vi "command_line_args.vi"(8 "error in (no error)":errorcluster, 10 "App.Args":string[](array[string]), 11 "Message Queues In":T1) -> (0 "error out":errorcluster, 2 "2D Array":string[][](array[string]), 3 "Message Queues Out":T1)   [LabVIEW 2013]
doc: "Receives the Command Line Arguments provided when the application was executed. The commands are decoded and translated to GUI sequence of GUI states for Main.vis"
uses:
  queues/que_all_message_queues.ctl
  queues/que_message_cluster.ctl
  type_def/general.ctl
  queues/que_enqueue_message_single.vi
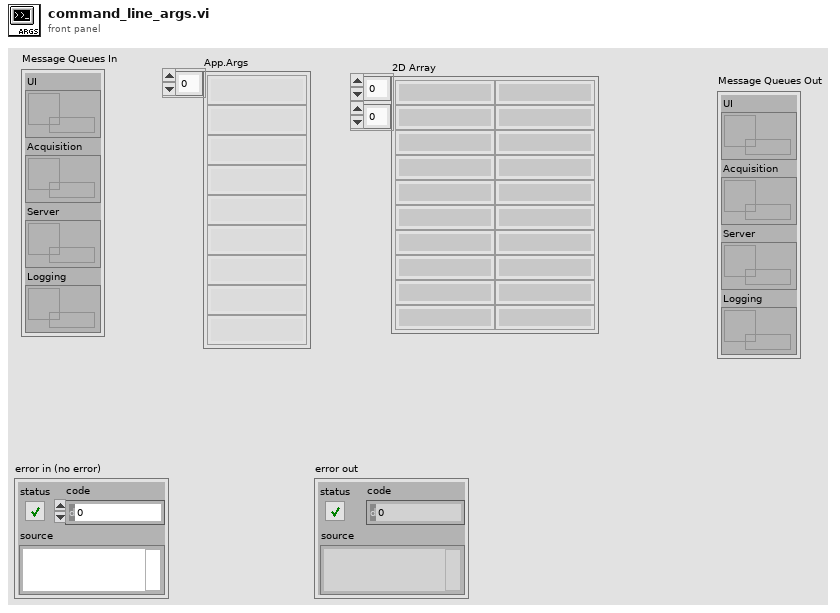
[diagram p1: front panel]
types:
  T1 = typedef "que_all_message_queues.ctl" = cluster{"UI":refnum<queue>, "Acquisition":refnum<queue>, "Server":refnum<queue>, "Logging":refnum<queue>}
  T2 = typedef "general.ctl" = cluster{"file_ext":string, "TCP port":i32, "#devices":i32, "log?":bool, "tcp?":bool, "language":string}
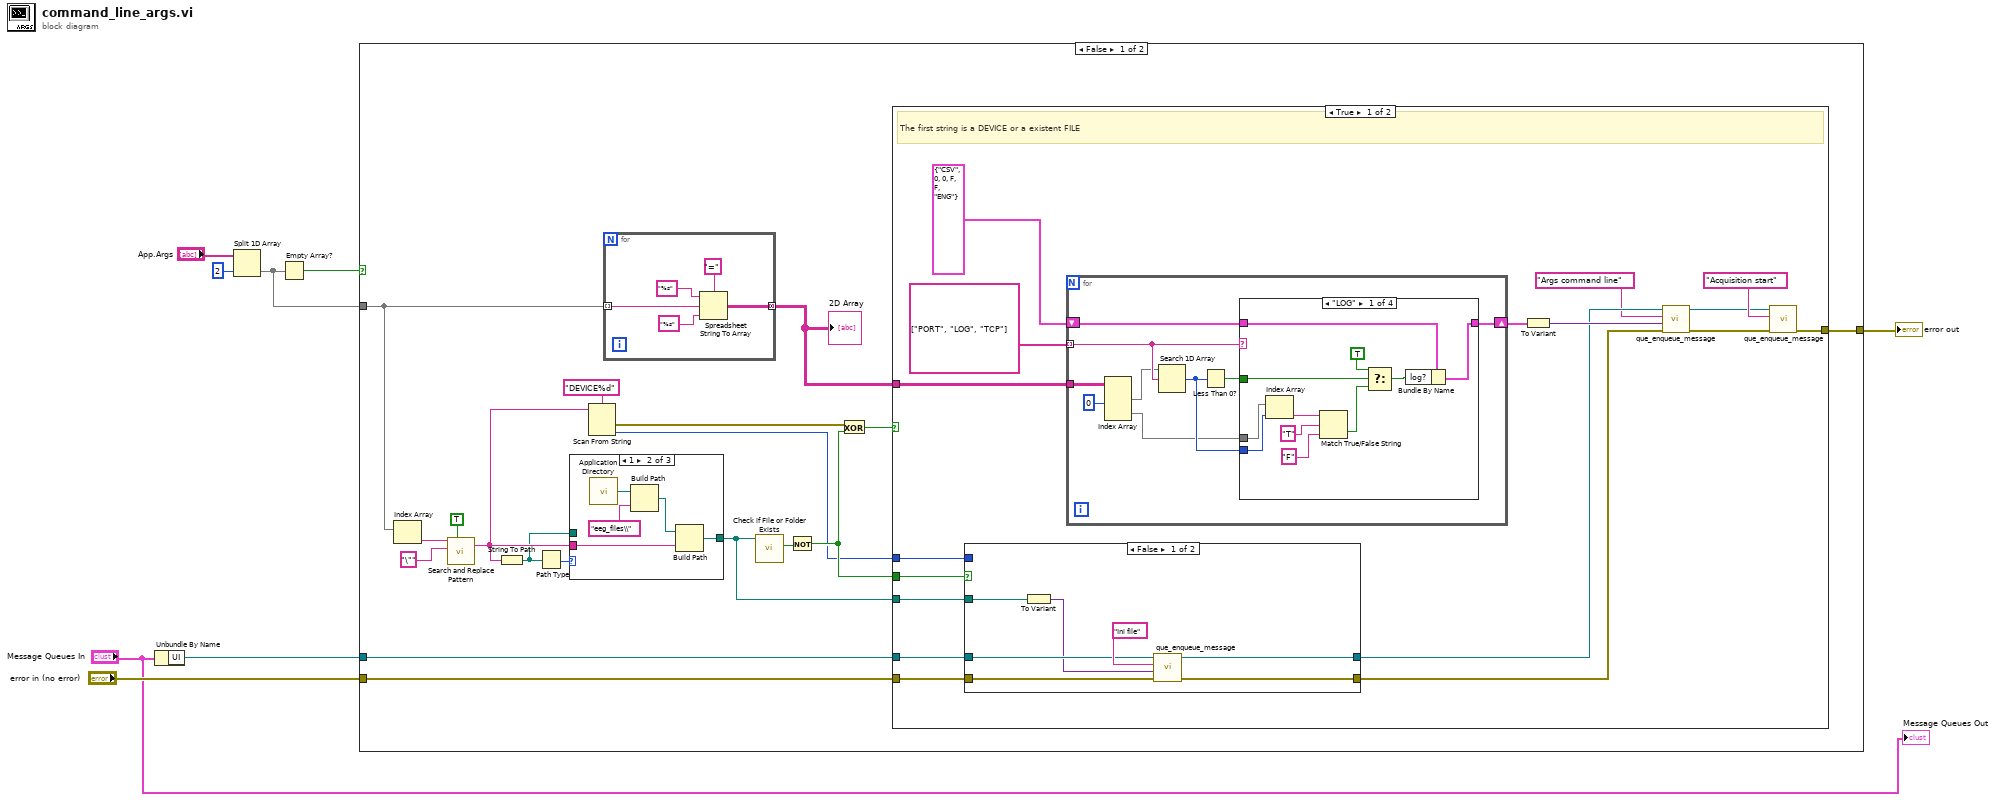
[diagram p0: block diagram]
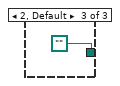
[diagram p3: hidden frame]
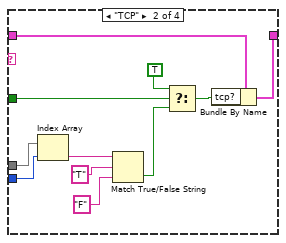
[diagram p4: hidden frame]
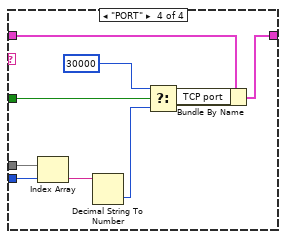
[diagram p6: hidden frame]
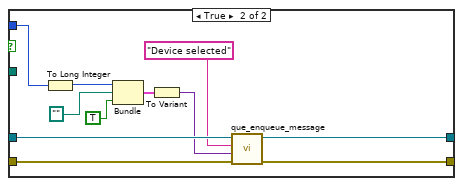
[diagram p7: hidden frame]
diagram:
  n1 = Unbundle By Name("Message Queues In") -> ("UI"=w2:refnum<queue>)
  n2 = Split 1D Array(array="App.Args", index=2) -> (second subarray=w4:string[])  [unwired: 1 out]
  n3 = Empty Array?(array=w4) -> (empty?=w5:bool)
  n4 = case shown="False" w5 {
    tunnel: [w26 w116] -> w8
    tunnel: "error in (no error)" -> [w9 w116]
    tunnel: w2 -> [w10 _]
    tunnel: w4 -> [w11 _]
    frame False {
      n5 = Index Array(array=w11) -> (element=w24:string)  [unwired: 1 in]
      n6 = call <vilib>:"Search and Replace Pattern.vi"("string"=w24, "regular expression (\"\")"="\"" ("regular expression (\"\")"), "replace all? (F)"=TRUE) -> ("result string"=w20:string)  [unwired: 2 in, 1 out]
      n7 = String To Path(string=w20) -> (path=w19:path)
      n8 = Path Type(1:w19) -> (0:w21:i16)
      n9 = case shown="1" w21 {
        tunnel: w20 -> [_ w32 _]
        tunnel: [w27 w28 path ""] -> w14
        tunnel: w19 -> [w27 _ _]
        frame 0 {
        }
        frame 1 {
          n10 = call <vilib>:"Application Directory.vi"() -> ("Application Directory"=w31:path)
          n11 = Build Path(base path=w31, name or relative path="eeg_files\\") -> (appended path=w29:path)
          n12 = Build Path(base path=w29, name or relative path=w32) -> (appended path=w28:path)
        }
        frame 2, Default {
        }
      }
      n13 = Scan From String(format string="DEVICE%d", input string=w20) -> (error out=w18:errorcluster, output 1=w13:i32)  [unwired: 3 in, 2 out]
      n14 = for {
        tunnel: w11 -> [w35] mode=indexing
        tunnel: [w34] -> w12 mode=concatenating
        n15 = Spreadsheet String To Array(delimiter (Tab)="=", format string="%s", spreadsheet string=w35, array type (2D Dbl)="%s" ("format string")) -> (array=w34:string[][])
      }
      "2D Array" <- w12
      n16 = call <vilib>:"Check if File or Folder Exists.vi"("path"=w14) -> ("file or folder exists?"=w17:bool)  [unwired: 8 in, 2 out]
      n17 = Not(x=w17) -> (.not. x?=w15:bool)
      n18 = Exclusive Or(1:w15, 2:w18) -> (0:w16:bool)
      n19 = case shown="True" w16 {
        tunnel: w9 -> [w40 w115]
        tunnel: [w46 w115] -> w26
        tunnel: w12 -> [w45 _]
        tunnel: w15 -> [w44 _]
        tunnel: w14 -> [w43 _]
        tunnel: w13 -> [w42 _]
        tunnel: w10 -> [w41 _]
        frame True {
          # "The first string is a DEVICE or a existent FILE"
          n20 = case shown="False" w44 {
            tunnel: w41 -> [w102 w114]
            tunnel: [w99 w108] -> w53
            tunnel: [w98 w107] -> w52
            tunnel: w40 -> [w97 w106]
            tunnel: w43 -> [w100 _]
            tunnel: w42 -> [_ w105]
            frame False {
              n21 = To Variant(anything=w100) -> (Variant=w101:variant)
              n22 = call-poly "que_enqueue_message.vi"("error in (no error)"=w97, "Message Data"=w101, "Message"="Ini file", "Message Queue"=w102) -> ("error out"=w98:errorcluster, "dup Message Queue"=w99:refnum<queue>)  [unwired: 6 in]
            }
            frame True {
              n23 = To Long Integer(number=w105) -> (32bit integer=w112:i32)
              n24 = Bundle(w112, path "", TRUE) -> (w111:cluster{i32, path, bool})  [unwired: 1 in]
              n25 = To Variant(anything=w111) -> (Variant=w110:variant)
              n26 = call-poly "que_enqueue_message.vi"("error in (no error)"=w106, "Message Data"=w110, "Message"="Device selected", "Message Queue"=w114) -> ("error out"=w107:errorcluster, "dup Message Queue"=w108:refnum<queue>)  [unwired: 6 in]
            }
          }
          n27 = for {
            tunnel: string[] ["PORT", "LOG", "TCP"] -> [w61] mode=indexing
            shift-right: [w63] -> w47
            shift-left: T2 {"file_ext"="CSV", "TCP port"=0, "#devices"=0, "log?"=FALSE, "tcp?"=FALSE, "language"="ENG"} ("general") -> [w62]
            tunnel: w45 -> [w58]
            n28 = Index Array(array=w58, index (col) #1=0 ("disabled index (col)")) -> (element #1=w57:string[], element #2=w56:string[])  [unwired: 3 in]
            n29 = Search 1D Array(1D array=w57, element=w61) -> (index of element=w64:i32)  [unwired: 1 in]
            n30 = Less Than 0?(x=w64) -> (x < 0?=w60:bool)
            n31 = case shown="\"LOG\"" w61 {
              tunnel: w64 -> [w65 w76 _ w92]
              tunnel: [w74 w85 w87 w95] -> w63
              tunnel: w62 -> [w75 w86 w87 w96]
              tunnel: w60 -> [w73 w84 _ w94]
              tunnel: w56 -> [w71 w82 _ w89]
              frame "LOG" {
                n32 = Index Array(array=w71, index=w65) -> (element=w70:string)
                n33 = Match True/False String(2:"F" ("false string"), 3:"T" ("true string"), 4:w70) -> (0:w67:bool)  [unwired: 1 out]
                n34 = Select(t=TRUE, s=w73, f=w67) -> (s? t:f=w66:bool)
                n35 = Bundle By Name(cluster=w75, "log?"=w66) -> (w74:T2)
              }
              frame "TCP" {
                n36 = Index Array(array=w82, index=w76) -> (element=w81:string)
                n37 = Match True/False String(2:"F" ("false string"), 3:"T" ("true string"), 4:w81) -> (0:w78:bool)  [unwired: 1 out]
                n38 = Select(t=TRUE, s=w84, f=w78) -> (s? t:f=w77:bool)
                n39 = Bundle By Name(cluster=w86, "tcp?"=w77) -> (w85:T2)
              }
              frame Default {
              }
              frame "PORT" {
                n40 = Index Array(array=w89, index=w92) -> (element=w88:string)
                n41 = Decimal String To Number(string=w88) -> (number=w91:i32)  [unwired: 2 in, 1 out]
                n42 = Select(t=30000 ("general.port"), s=w94, f=w91) -> (s? t:f=w90:i32)
                n43 = Bundle By Name(cluster=w96, "TCP port"=w90) -> (w95:T2)
              }
            }
          }
          n44 = To Variant(anything=w47) -> (Variant=w54:variant)
          n45 = call-poly "que_enqueue_message.vi"("error in (no error)"=w52, "Message Data"=w54, "Message"="Args command line", "Message Queue"=w53) -> ("error out"=w48:errorcluster, "dup Message Queue"=w49:refnum<queue>)  [unwired: 6 in]
          n46 = call-poly "que_enqueue_message.vi"("error in (no error)"=w48, "Message"="Acquisition start", "Message Queue"=w49) -> ("error out"=w46:errorcluster)  [unwired: 7 in, 1 out]
        }
        frame False {
          # "The first string in not a DEVICE nor a existent FILE"
        }
      }
    }
    frame True {
    }
  }
  "error out" <- w8
  "Message Queues Out" <- "Message Queues In"
